vi "getConnectionPoint.vi"(0 "reference":refnum<class "ChoiceNode.lvclass">, 1 "direction":refnum<class "Direction.lvclass">, 5 "error in (no error)":errorcluster) -> (14 "reference out":refnum<class "ChoiceNode.lvclass">, 15 "point2D":T1 {"y" format="%.2f"; "x" format="%.2f"}, 19 "error out":errorcluster)   [LabVIEW 2016, in "ChoiceNode.lvclass"]
doc: "getConnectionPoint"
uses:
  <resource>/Framework/Providers/Open_GDS/UML/ChoiceNode_class/ChoiceNode.lvclass
  C:/Program Files (x86)/National Instruments/LabVIEW 2016/resource/Framework/Providers/Open_GDS/UML/RectangularNode_class/RectangularNode.lvclass
  <resource>/Framework/Providers/Open_GDS/UML/Direction_class/Direction.lvclass
  <resource>/Framework/Providers/Open_GDS/UML/General/Point/Point Point2D.ctl
  <resource>/Framework/Providers/Open_GDS/UML/RectangularNode_class/RectangularNode.lvclass
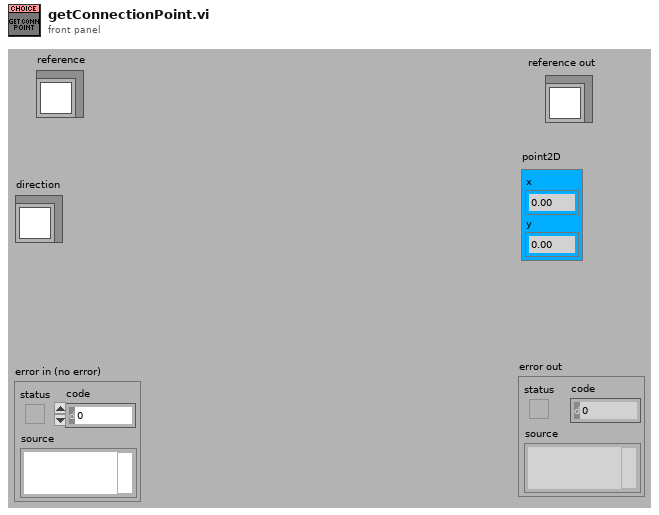
[diagram p1: front panel]
types:
  T1 = typedef "Point Point2D.ctl" = cluster{"x":dbl, "y":dbl}
  T2 = typedef "RectangularNode.lvclass/ObjectAttributes.ctl" = cluster{"bounds":T3}
  T3 = typedef "Rectangle Rectangle2D.ctl" = cluster{"x":dbl, "y":dbl, "width":dbl, "height":dbl}
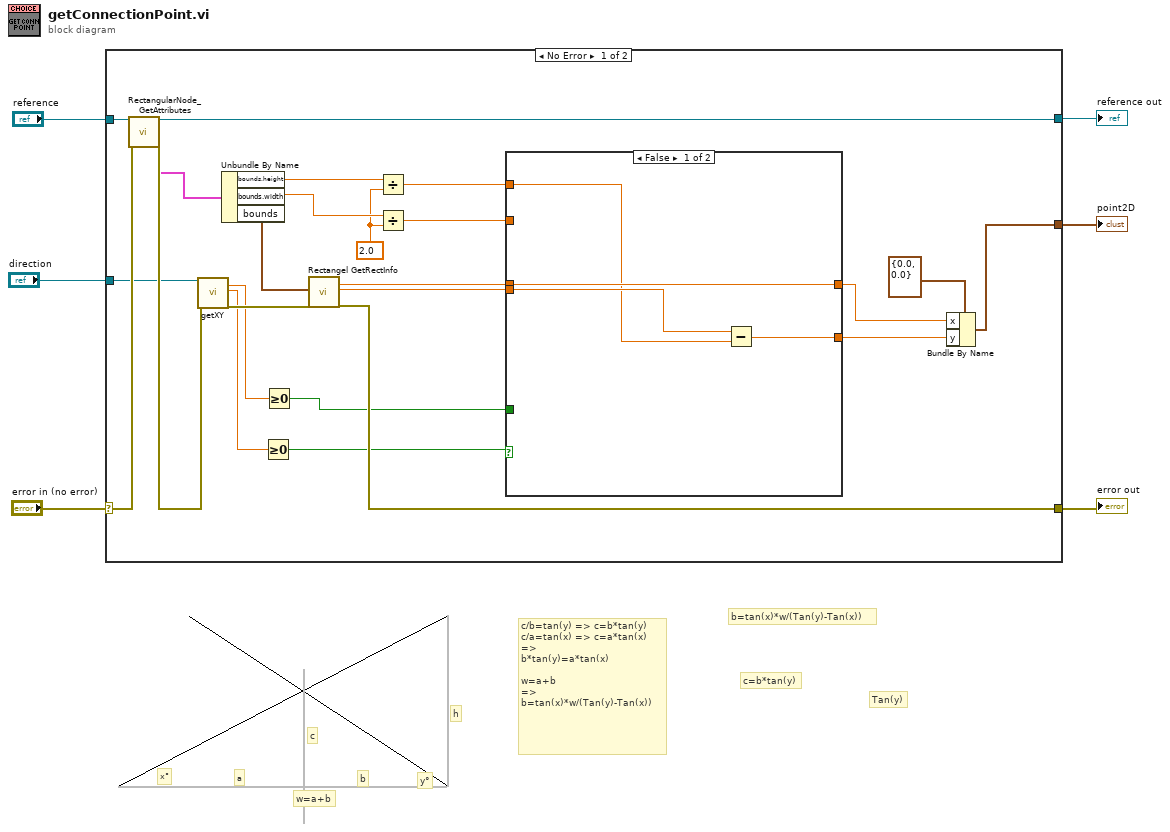
[diagram p0: block diagram]
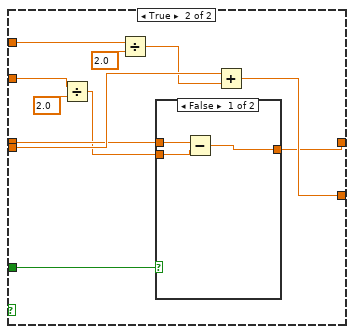
[diagram p2: hidden frame]
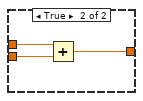
[diagram p3: hidden frame]
diagram:
  # "Tan(y)"
  # "c=b*tan(y)"
  # "b=tan(x)*w/(Tan(y)-Tan(x))"
  # "c/b=tan(y) => c=b*tan(y)\nc/a=tan(x) => c=a*tan(x)\n=>\nb*tan(y)=a*tan(x)\n\nw=a+b\n=>\nb=tan(x)*w/(Tan(y)-Tan(x))"
  # "c"
  # "y°"
  # "x°"
  # "h"
  # "w=a+b"
  # "b"
  # "a"
  n1 = case shown="No Error" "error in (no error)" {
    selector: "error in (no error)" -> [w30 w52]
    tunnel: "reference" -> [w29 w53]
    tunnel: [w21 w52] -> w4
    tunnel: [w8 w53] -> w3
    tunnel: "direction" -> [w20 _]
    tunnel: [w9 _] -> w1
    frame No Error {
      w25 = 2.0 ("y")
      n2 = call <resource>:"RectangularNode_GetAttributes.vi"("reference in"=w29, "error in (no error)"=w30) -> ("reference out"=w8:refnum<class "ChoiceNode.lvclass">, "Data"=w7:T2, "error out"=w28:errorcluster)  [unwired: 14 in, 1 out]
      n3 = call <resource>:"getXY.vi"("reference"=w20, "error in (no error)"=w28) -> ("x"=w18:dbl, "y"=w19:dbl, "error out"=w24:errorcluster)  [unwired: 15 out]
      n4 = Unbundle By Name(w7) -> ("bounds.height"=w27:dbl, "bounds.width"=w26:dbl, "bounds"=w23:T3)
      n5 = Greater Or Equal To 0?(x=w19) -> (x >= 0?=w17:bool)
      n6 = Greater Or Equal To 0?(x=w18) -> (x >= 0?=w10:bool)
      n7 = call <resource>:"Rectangel GetRectInfo.vi"("bounds"=w23, "error in (no error)"=w24) -> ("centerX"=w16:dbl, "centerY"=w13:dbl, "error out"=w21:errorcluster)  [unwired: 15 out]
      n8 = Divide(x=w27, y=w25) -> (x/y=w12:dbl)
      n9 = Divide(x=w26, y=w25) -> (x/y=w15:dbl)
      n10 = case shown="False" w17 {
        tunnel: w16 -> [w34 w37]
        tunnel: w15 -> [_ w38]
        tunnel: [w34 w35] -> w14
        tunnel: w13 -> [w33 w44]
        tunnel: w12 -> [w32 w43]
        tunnel: [w31 w40] -> w11
        tunnel: w10 -> [_ w45]
        frame False {
          n11 = Subtract(x=w33, y=w32) -> (x-y=w31:dbl)
        }
        frame True {
          n12 = Divide(x=w38, y=2.0) -> (x/y=w36:dbl)
          n13 = Divide(x=w43, y=2.0) -> (x/y=w41:dbl)
          n14 = case shown="False" w45 {
            tunnel: w37 -> [w48 w51]
            tunnel: w36 -> [w47 w50]
            tunnel: [w46 w49] -> w35
            frame False {
              n15 = Subtract(x=w48, y=w47) -> (x-y=w46:dbl)
            }
            frame True {
              n16 = Add(x=w51, y=w50) -> (x+y=w49:dbl)
            }
          }
          n17 = Add(x=w44, y=w41) -> (x+y=w40:dbl)
        }
      }
      n18 = Bundle By Name(cluster=T1 {"x"=0.0, "y"=0.0} ("point2D"), "x"=w14, "y"=w11) -> (w9:T1)
    }
    frame Error {
    }
  }
  "reference out" <- w3
  "error out" <- w4
  "point2D" <- w1
